vi "Verify.vi"(8 "error in (no error)":errorcluster, 11 "Mock in":refnum<class "Mock.lvclass">) -> (0 "error out":errorcluster, 1 "Errors":errorcluster[](array[cluster]), 2 "Results":cluster{"Passed?":bool, "Message":string}[](array[cluster]))   [LabVIEW 2020, in "Mock.lvclass"]
uses:
  Mock.lvclass
  Mock.lvclass/Mock.ctl
  Expectation/Expectation.lvclass
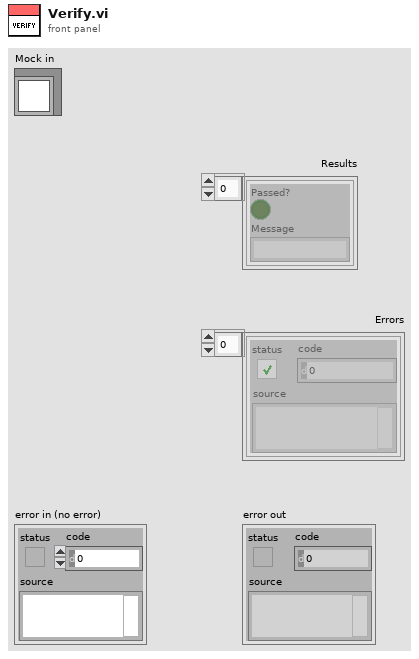
[diagram p1: front panel]
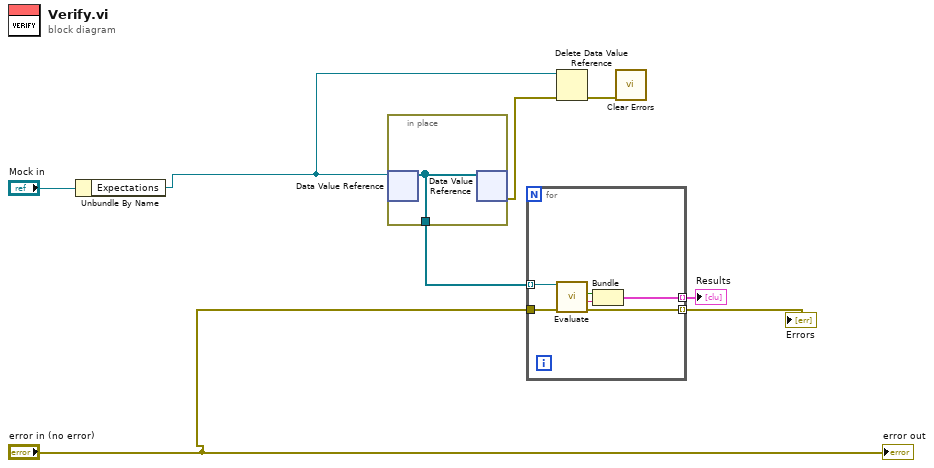
[diagram p0: block diagram]
diagram:
  n1 = Unbundle By Name("Mock in") -> ("Expectations"=w2:refnum<data-value>)
  n2 = in-place {
    in-place-border: [w9] -> w3
    n3 = in-place-dvr #1(w2) -> (w9:refnum<class "Expectation.lvclass">[])  [unwired: 1 out]
    n4 = in-place-dvr #1(w9) -> (w1:errorcluster)  [unwired: 1 out]
  }
  n5 = for {
    tunnel: "error in (no error)" -> [w15]
    tunnel: [w14] -> w6 mode=indexing
    tunnel: w3 -> [w13] mode=indexing
    tunnel: [w10] -> w5 mode=indexing
    n6 = call-dynamic "Evaluate.vi"("error in (no error)"=w15, "Expectation in"=w13) -> ("error out"=w14:errorcluster, "Message"=w11:string, "Passed?"=w12:bool)  [unwired: 7 in]
    n7 = Bundle("Passed?"=w12, "Message"=w11) -> (w10:cluster{"Passed?":bool, "Message":string})  [unwired: 1 in]
  }
  "Errors" <- w6
  "Results" <- w5
  n8 = Delete Data Value Reference(data value reference=w2, error in=w1) -> (error out=w4:errorcluster)  [unwired: 1 out]
  n9 = call <vilib>:"Clear Errors.vi"("error in (no error)"=w4) -> ()  [unwired: 5 in, 2 out]
  "error out" <- "error in (no error)"
